vi "test Get Status Messages.vi"(8 "error in":errorcluster, 11 "TestCase in":refnum<class "Scripting.lvclass">) -> (0 "error out":errorcluster, 3 "TestCase out":refnum<class "Scripting.lvclass">)   [LabVIEW 2020, in "Scripting.lvclass"]
uses:
  Scripting.lvclass
  C:/Git/niveristand-custom-device-testing-tools/VeriStandScriptingTestCase/VeriStandScriptingTestCase.lvclass
  Shared/1553 Channel.ctl
  Shared/Address.ctl
  Shared/Message Definition.ctl
  Shared/Message Type.ctl
  Shared/Terminal Endpoint.ctl
  Shared/Parameter Definition.ctl
  niveristand-custom-device-testing-tools/VeriStandScriptingTestCase/VeriStandScriptingTestCase.lvclass/VeriStandScriptingTestCase.ctl
  niveristand-custom-device-testing-tools/VeriStandScriptingTestCase/Read Target.vi
  NationalInstruments.VeriStand.SystemDefinitionAPI
  <vilib>/addons/_JKI Toolkits/VI Tester/TestCase.llb/TestCase.lvclass
  Scripting/Ballard MIL-STD-1553 Scripting.lvlib
  C:/Program Files (x86)/National Instruments/LabVIEW 2020/vi.lib/addons/_JKI Toolkits/VI Tester/TestCase.llb/TestCase.lvclass
  C:/Git/niveristand-ballard-milStd1553-custom-device/Source/Custom Device Support/Tests/Unit/Scripting/Scripting.lvclass
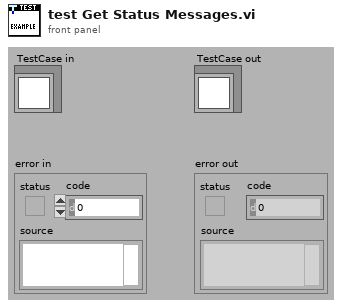
[diagram p1: front panel]
types:
  T1 = typedef "1553 Channel.ctl" = cluster{"HW channel":u16, "terminal addresses":T2[], "acyclic frame names":string[], "messages":T3[]}
  T2 = typedef "Address.ctl" = u16
  T3 = typedef "Message Definition.ctl" = cluster{"name":string, "message type":T4, "endpoint Tx":T5, "endpoint Rx":T5, "create timestamp channel":bool, "mode code":u16, "number of words":u16, "parameters":cluster{"name":string, "default value":dbl, "unit":string, "parameter definition":T6}[]}
  T4 = typedef "Message Type.ctl" = string
  T5 = typedef "Terminal Endpoint.ctl" = cluster{"terminal address":T2, "subaddress":T2}
  T6 = typedef "Parameter Definition.ctl" = cluster{"start index":i32, "size (bits)":i32, "encoding":enum16{"BNR", "BCD", "Discrete"}, "signed":bool, "multiplier":dbl, "offset":dbl}
  T7 = typedef "Custom Device API.lvlib/Custom Device Item Ref.ctl" = u64
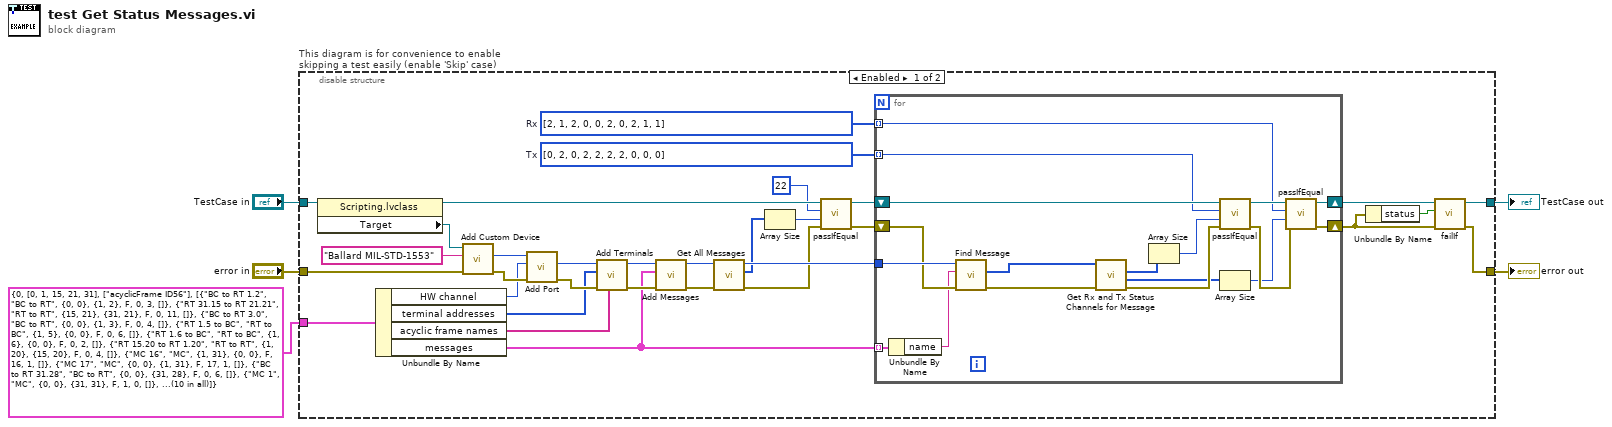
[diagram p0: block diagram]
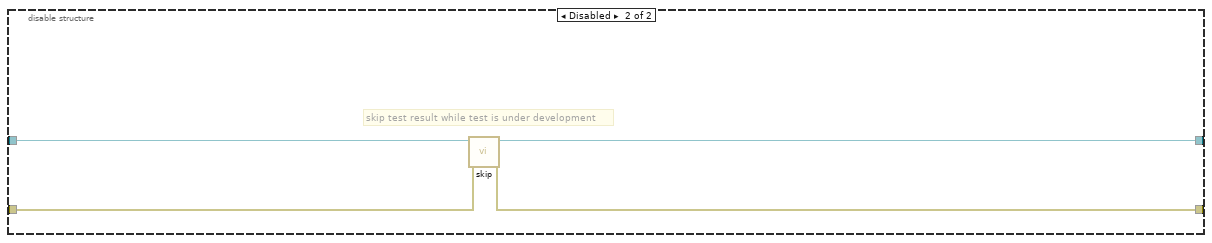
[diagram p2: hidden frame]
diagram:
  n1 = disable-structure "This diagram is for convenience to enable skipping a test easily (enable 'Skip' case)" shown="Enabled" {
    disable-tunnel: "TestCase in" -> [w35 w59]
    disable-tunnel: [w32 w57] -> w2
    disable-tunnel: [w33 w58] -> w4
    disable-tunnel: "error in" -> [w37 w56]
    disable-tunnel: T1 {"HW channel"=0, "terminal addresses"=[0, 1, 15, 21, 31], "acyclic frame names"=["acyclicFrame ID56"], "messages"=[{"name"="BC to RT 1.2", "message type"="BC to RT", "endpoint Tx"={"terminal address"=0, "subaddress"=0}, "endpoint Rx"={"terminal address"=1, "subaddress"=2}, "create timestamp channel"=FALSE, "mode code"=0, "number of words"=3, "parameters"=[]}, {"name"="RT 31.15 to RT 21.21", "message type"="RT to RT", "endpoint Tx"={"terminal address"=15, "subaddress"=21}, "endpoint Rx"={"terminal address"=31, "subaddress"=21}, "create timestamp channel"=FALSE, "mode code"=0, "number of words"=11, "parameters"=[]}, {"name"="BC to RT 3.0", "message type"="BC to RT", "endpoint Tx"={"terminal address"=0, "subaddress"=0}, "endpoint Rx"={"terminal address"=1, "subaddress"=3}, "create timestamp channel"=FALSE, "mode code"=0, "number of words"=4, "parameters"=[]}, {"name"="RT 1.5 to BC", "message type"="RT to BC", "endpoint Tx"={"terminal address"=1, "subaddress"=5}, "endpoint Rx"={"terminal address"=0, "subaddress"=0}, "create timestamp channel"=FALSE, "mode code"=0, "number of words"=6, "parameters"=[]}, {"name"="RT 1.6 to BC", "message type"="RT to BC", "endpoint Tx"={"terminal address"=1, "subaddress"=6}, "endpoint Rx"={"terminal address"=0, "subaddress"=0}, "create timestamp channel"=FALSE, "mode code"=0, "number of words"=2, "parameters"=[]}, {"name"="RT 15.20 to RT 1.20", "message type"="RT to RT", "endpoint Tx"={"terminal address"=1, "subaddress"=20}, "endpoint Rx"={"terminal address"=15, "subaddress"=20}, "create timestamp channel"=FALSE, "mode code"=0, "number of words"=4, "parameters"=[]}, {"name"="MC 16", "message type"="MC", "endpoint Tx"={"terminal address"=1, "subaddress"=31}, "endpoint Rx"={"terminal address"=0, "subaddress"=0}, "create timestamp channel"=FALSE, "mode code"=16, "number of words"=1, "parameters"=[]}, {"name"="MC 17", "message type"="MC", "endpoint Tx"={"terminal address"=0, "subaddress"=0}, "endpoint Rx"={"terminal address"=1, "subaddress"=31}, "create timestamp channel"=FALSE, "mode code"=17, "number of words"=1, "parameters"=[]}, {"name"="BC to RT 31.28", "message type"="BC to RT", "endpoint Tx"={"terminal address"=0, "subaddress"=0}, "endpoint Rx"={"terminal address"=31, "subaddress"=28}, "create timestamp channel"=FALSE, "mode code"=0, "number of words"=6, "parameters"=[]}, {"name"="MC 1", "message type"="MC", "endpoint Tx"={"terminal address"=0, "subaddress"=0}, "endpoint Rx"={"terminal address"=31, "subaddress"=31}, "create timestamp channel"=FALSE, "mode code"=1, "number of words"=0, "parameters"=[]}]} ("1553 channel") -> [w9 _]
    frame Enabled {
      w6 = i32[] [2, 1, 2, 0, 0, 2, 0, 2, 1, 1]  # Rx
      w7 = i32[] [0, 2, 0, 2, 2, 2, 2, 0, 0, 0]  # Tx
      n2 = property class="Scripting.lvclass"(reference=w35) -> (reference out=w19:refnum<class "Scripting.lvclass">, "Target"=w34:refnum<k24>)  [unwired: 1 in, 1 out]
      n3 = Unbundle By Name(w9) -> ("HW channel"=w27:u16, "terminal addresses"=w22:T2[], "acyclic frame names"=w21:string[], "messages"=w16:T3[])
      n4 = call "Add Custom Device.vi"("error in"=w37, "name"="Ballard MIL-STD-1553", "target in"=w34) -> ("error out"=w30:errorcluster, "Ballard MIL-STD 1553 custom device"=w29:T7)  [unwired: 6 in, 1 out]
      n5 = call "Add Port.vi"("error in"=w30, "port number"=w27, "Ballard MIL-STD 1553 custom device in"=w29) -> ("error out"=w25:errorcluster, "port"=w26:T7)  [unwired: 6 in, 1 out]
      n6 = call "Add Terminals.vi"("acyclic frame names"=w21, "error in"=w25, "terminal addresses"=w22, "port in"=w26) -> ("error out"=w23:errorcluster, "port out"=w24:T7)  [unwired: 6 in]
      n7 = call "Add Messages.vi"("error in"=w23, "messages"=w16, "port in"=w24) -> ("error out"=w20:errorcluster, "port out"=w28:T7)  [unwired: 7 in]
      n8 = call "Get All Messages.vi"("error in"=w20, "port in"=w28) -> ("error out"=w14:errorcluster, "messages"=w12:T7[], "port out"=w17:T7)  [unwired: 7 in]
      n9 = Array Size(array=w12) -> (size(s)=w18:i32)
      n10 = call-dynamic "passIfEqual.vi"("error in (no error)"=w14, "y"=w18, "x"=22 ("size(s)"), "TestCase in"=w19) -> ("error out"=w13:errorcluster, "TestCase out"=w10:refnum<class "Scripting.lvclass">)  [unwired: 6 in]
      n11 = for {
        shift-right: [w49] -> w8
        shift-left: w13 -> [w54]
        tunnel: w16 -> [w53] mode=indexing
        shift-right: [w50] -> w11
        shift-left: w10 -> [w48]
        tunnel: w17 -> [w55]
        tunnel: w7 -> [w42] mode=indexing
        tunnel: w6 -> [w38] mode=indexing
        n12 = Unbundle By Name(w53) -> ("name"=w45:string)
        n13 = call "Find Message.vi"("error in"=w54, "message name"=w45, "port in"=w55) -> ("error out"=w52:errorcluster, "message refs"=w43:T7[])  [unwired: 5 in, 2 out]
        n14 = call "Get Rx and Tx Status Channels for Message.vi"("error in"=w52, "message refs"=w43) -> ("error out"=w44:errorcluster, "Rx status channels"=w40:T7[], "Tx status channels"=w46:T7[])  [unwired: 6 in, 1 out]
        n15 = Array Size(array=w46) -> (size(s)=w41:i32)
        n16 = call-dynamic "passIfEqual.vi"("error in (no error)"=w44, "y"=w41, "x"=w42, "TestCase in"=w48) -> ("error out"=w51:errorcluster, "TestCase out"=w47:refnum<class "Scripting.lvclass">)  [unwired: 6 in]
        n17 = Array Size(array=w40) -> (size(s)=w39:i32)
        n18 = call-dynamic "passIfEqual.vi"("error in (no error)"=w51, "y"=w39, "x"=w38, "TestCase in"=w47) -> ("error out"=w49:errorcluster, "TestCase out"=w50:refnum<class "Scripting.lvclass">)  [unwired: 6 in]
      }
      n19 = Unbundle By Name(w8) -> ("status"=w31:bool)
      n20 = call-dynamic "failIf.vi"("error in (no error)"=w8, "fail"=w31, "TestCase in"=w11) -> ("error out"=w33:errorcluster, "TestCase out"=w32:refnum<class "Scripting.lvclass">)  [unwired: 7 in]
    }
    frame Disabled {
      # "skip test result while test is under development"
      n21 = call <vilib>:"skip.vi"("error in (no error)"=w56, "TestCase in"=w59) -> ("error out"=w58:errorcluster, "TestCase out"=w57:refnum<class "Scripting.lvclass">)  [unwired: 8 in]
    }
  }
  "error out" <- w4
  "TestCase out" <- w2
